vi "DidStop.vi"(6 "Wait for Module to stop?":bool, 7 "Exit via Stop Module Req?":bool, 8 "error in (no error)":errorcluster, 11 "ModuleAdmin":refnum<class "ModuleAdmin.lvclass">) -> (0 "error out":errorcluster, 3 "ModuleAdmin":refnum<class "ModuleAdmin.lvclass">)   [LabVIEW 2014, in "DigitizerModule.lvlib"]
uses:
  DigitizerModule.lvlib
  <userlib>/NIST/ModuleAdminLib/ModuleAdmin/ModuleAdmin.lvclass
  PublicAPI/Arguments/Requests/clStopArgument.ctl
  clEventType.ctl
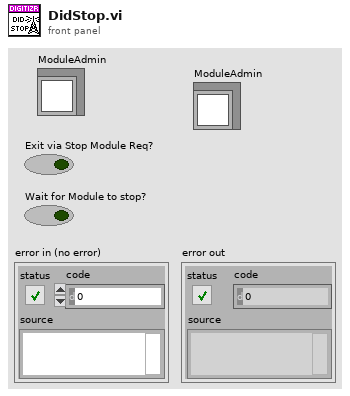
[diagram p1: front panel]
types:
  T1 = typedef "DigitizerModule.lvlib/clEventType.ctl" = cluster{"ModuleID":i32, "Data":variant}
  T2 = typedef "DigitizerModule.lvlib/clStopArgument.ctl" = cluster{"Exit via Stop Module Req?":bool, "Wait for Module to stop?":bool, "ModuleAdmin":refnum<class "ModuleAdmin.lvclass">}
  T3 = typedef "DigitizerModule.lvlib/clBroadcastEvents.ctl" = cluster{"DidInit":refnum<user-event>, "StatusUpdate":refnum<user-event>, "ErrorReport":refnum<user-event>, "DidStop":refnum<user-event>, "PathToINI":refnum<user-event>, "Channels":refnum<user-event>, "Acq":refnum<user-event>, "Trigger":refnum<user-event>, "Waveforms":refnum<user-event>}
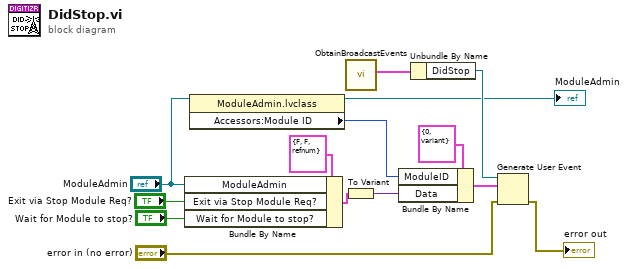
[diagram p0: block diagram]
diagram:
  n1 = Bundle By Name(cluster=T2 {"Exit via Stop Module Req?"=FALSE, "Wait for Module to stop?"=FALSE, "ModuleAdmin"=refnum} ("Stop Argument"), "ModuleAdmin"="ModuleAdmin", "Exit via Stop Module Req?"="Exit via Stop Module Req?", "Wait for Module to stop?"="Wait for Module to stop?") -> (w12:T2)
  n2 = property class="ModuleAdmin.lvclass"(reference="ModuleAdmin") -> (reference out=→"ModuleAdmin":refnum<class "ModuleAdmin.lvclass">, "Accessors:Module ID"=w2:i32)  [unwired: 1 in, 1 out]
  n3 = call "ObtainBroadcastEvents.vi"() -> ("clDigitizerBdcstEvents"=w13:T3)  [unwired: 10 in, 1 out]
  n4 = To Variant(anything=w12) -> (Variant=w9:variant)
  n5 = Bundle By Name(cluster=T1 {"ModuleID"=0, "Data"=variant} ("clBroadcast"), "ModuleID"=w2, "Data"=w9) -> (w8:T1)
  n6 = Unbundle By Name(w13) -> ("DidStop"=w11:refnum<user-event>)
  n7 = Generate User Event(user event=w11, event data cluster=w8, error in="error in (no error)") -> (error out=→"error out":errorcluster)  [unwired: 1 in, 1 out]
